vi "SLM Control.vi"() -> ()   [LabVIEW 2018]
uses:
  Controls/General Setting.ctl
  Controls/Buttons/Running Button.ctl
  Controls/Holo Setting.ctl
  Controls/Zernike Polynominals.ctl
  Controls/Buttons/Save Button.ctl
  Controls/Buttons/Load Button.ctl
  <vilib>/Utility/xml.llb/Read From XML File(string).vi
  <vilib>/Utility/xml.llb/Write to XML File(string).vi
panel:
  in  "Exit":bool
  in  "Load":T1
  in  "Save":T2
  in  "Holo 1 (Doughnut)":T3
  in  "Holo 0 (Z)":T3
  in  "General Setting":T6 {"Mode Matrix" items=["Name", "Sequence"]}
  out "Intensity Graph":u8[][](graph)
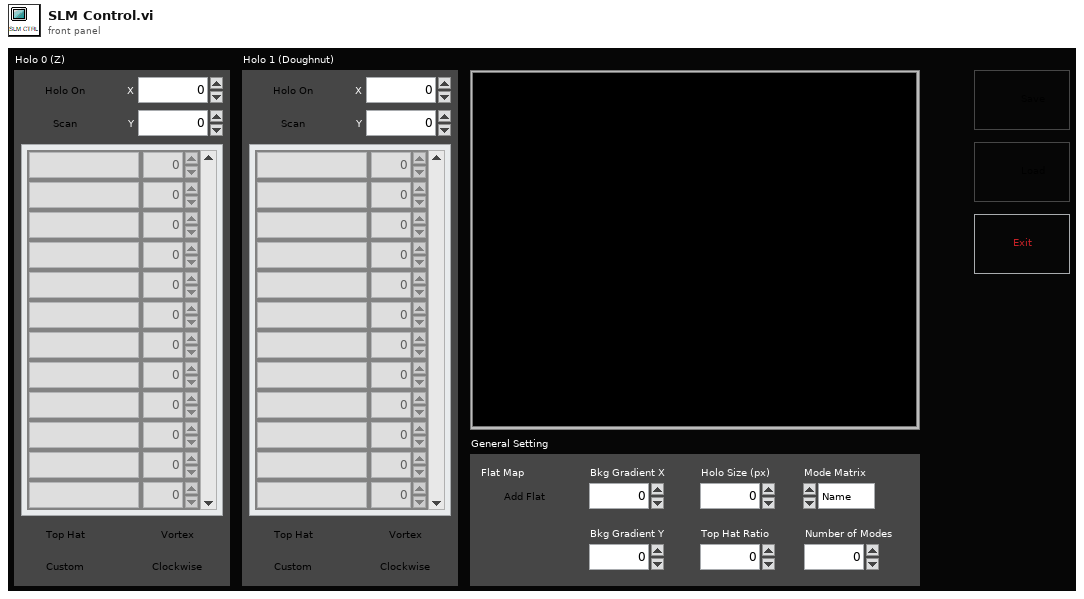
[diagram p1: front panel]
types:
  T1 = typedef "Load Button.ctl" = bool
  T2 = typedef "Save Button.ctl" = bool
  T3 = typedef "Holo Setting.ctl" = cluster{"Holo On":T4, "Scan":T4, "X":i16, "Y":i16, "Zernike Polynominals":T5, "Top Hat":T4, "Vortex":T4, "Clockwise":T4, "Custom":T4}
  T4 = typedef "Running Button.ctl" = bool
  T5 = typedef "Zernike Polynominals.ctl" = cluster{"Aberration Name":string, "Numeric":dbl}[]
  T6 = typedef "General Setting.ctl" = cluster{"Flat Map":T4, "Bkg Gradient X":dbl, "Bkg Gradient Y":dbl, "Holo Size (px)":i32, "Top Hat Ratio":dbl, "Number of Modes":i8, "Mode Matrix":u16}
  T7 = cluster{"Flat Map":T4, "Bkg Gradient X":bool, "Bkg Gradient Y":bool, "Holo Size (px)":bool, "Top Hat Ratio":bool, "Number of Modes":bool, "Mode Matrix":bool}
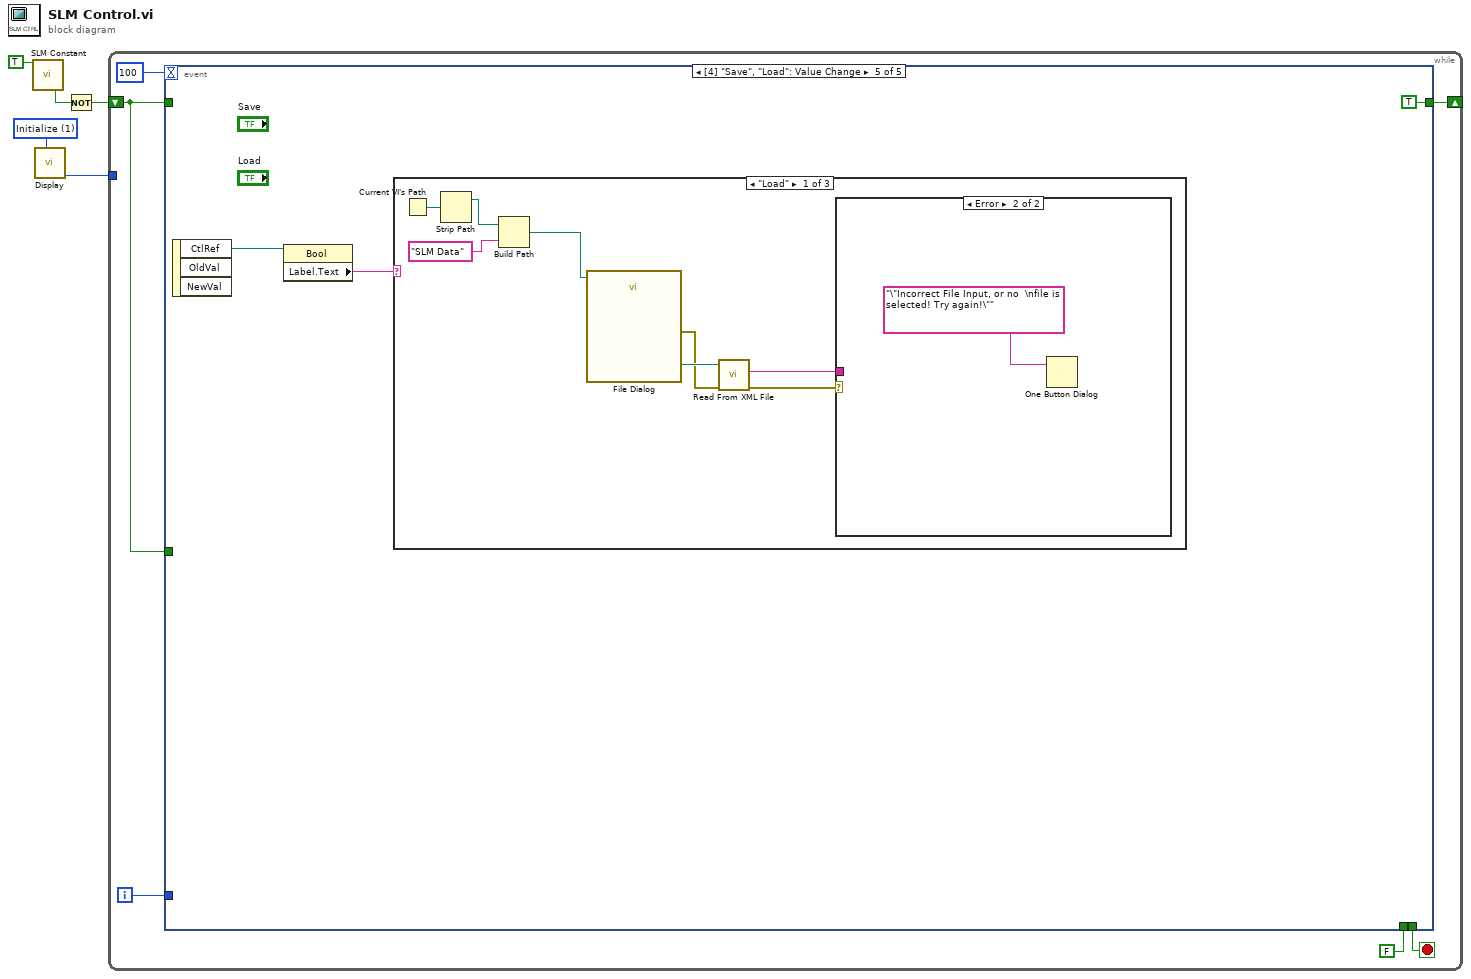
[diagram p0: block diagram]
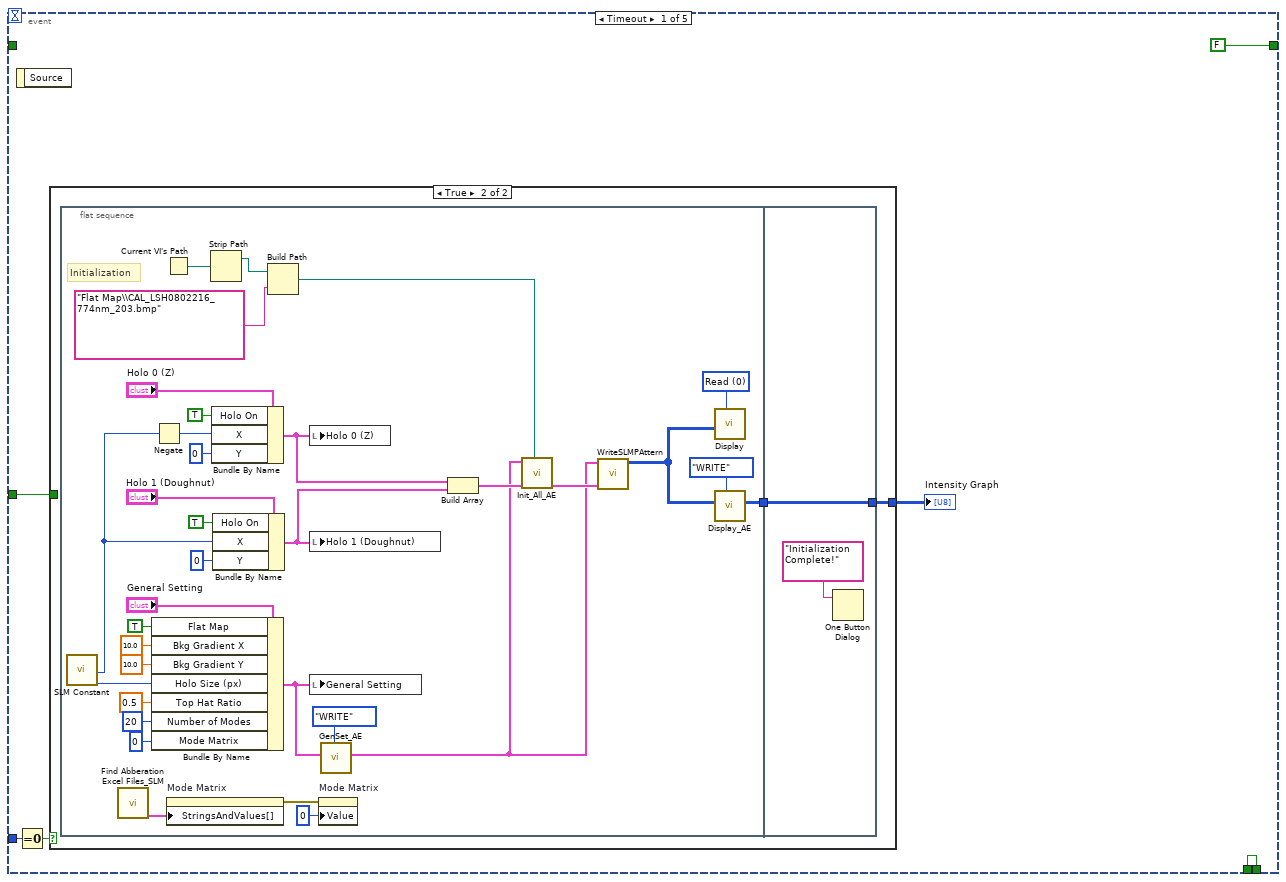
[diagram p2: hidden frame]
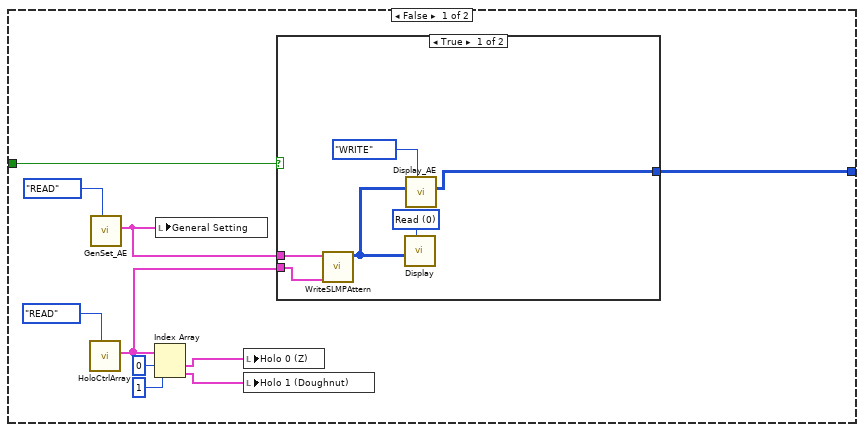
[diagram p3: hidden frame]
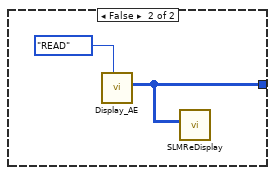
[diagram p4: hidden frame]
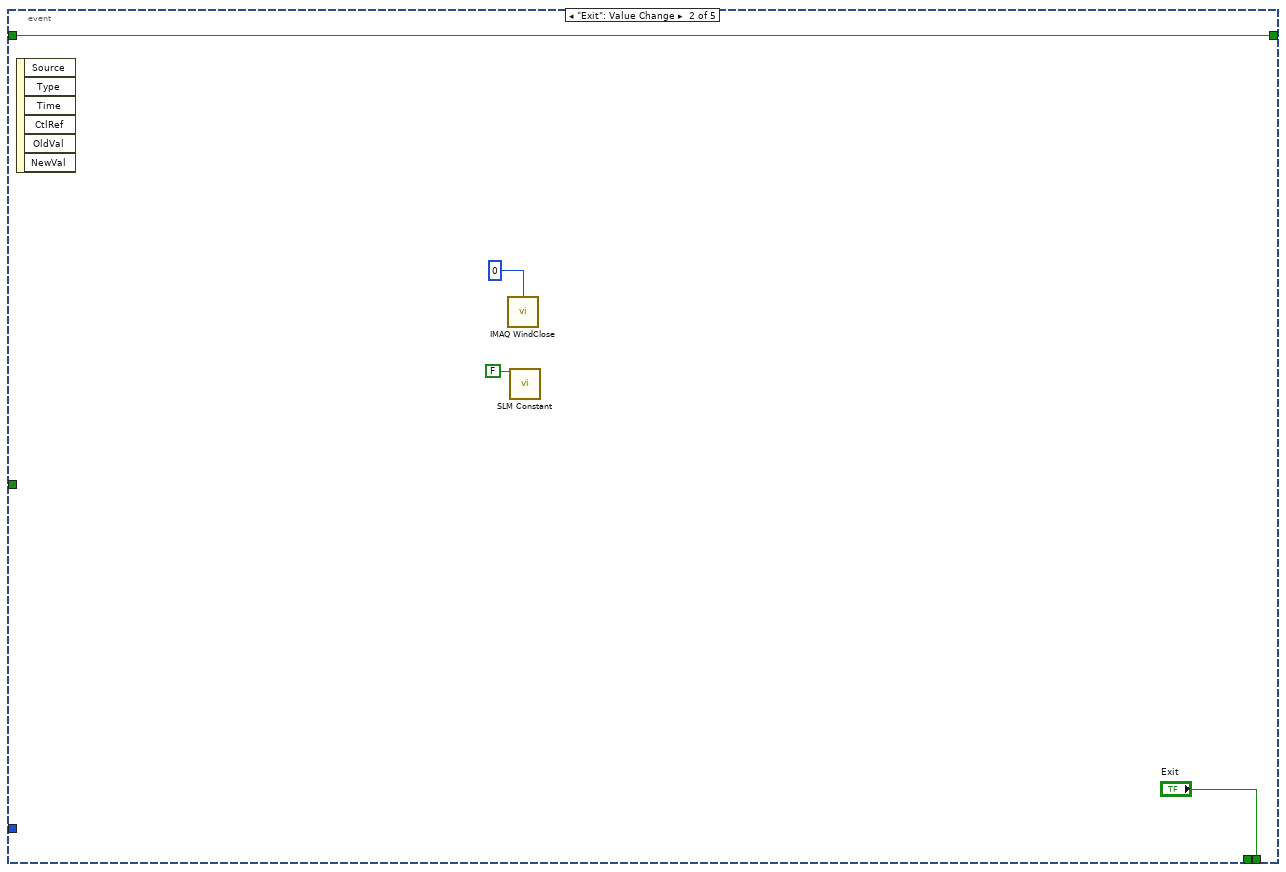
[diagram p5: hidden frame]
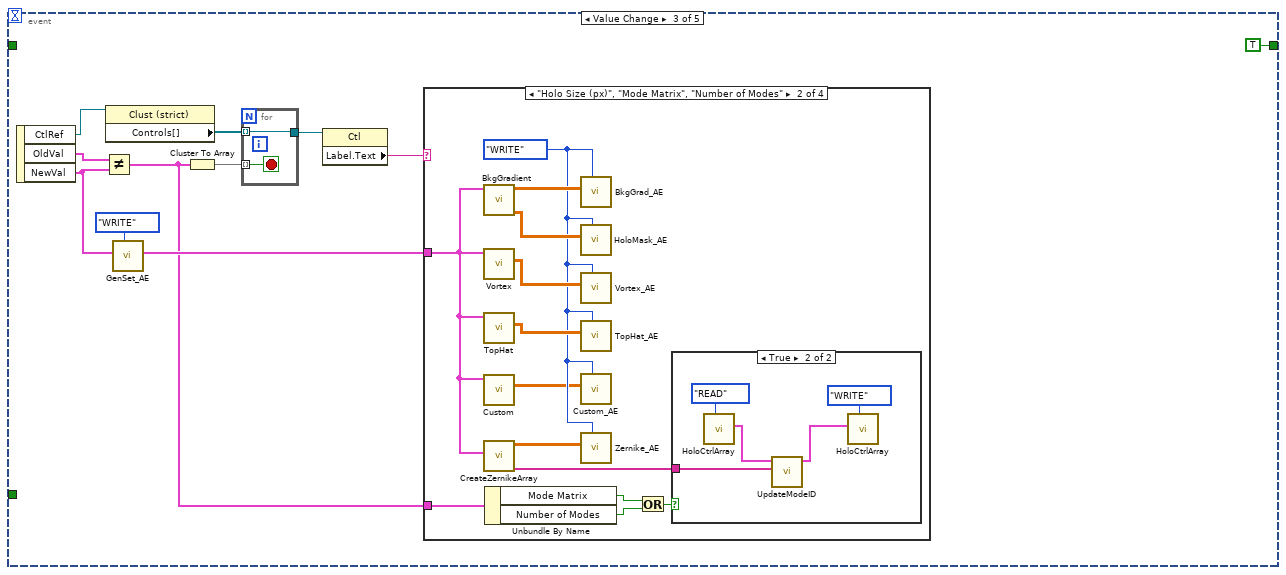
[diagram p6: hidden frame]
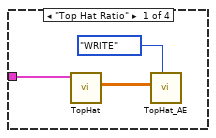
[diagram p7: hidden frame]
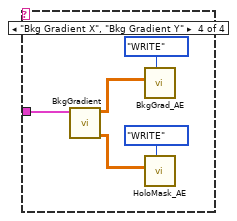
[diagram p10: hidden frame]
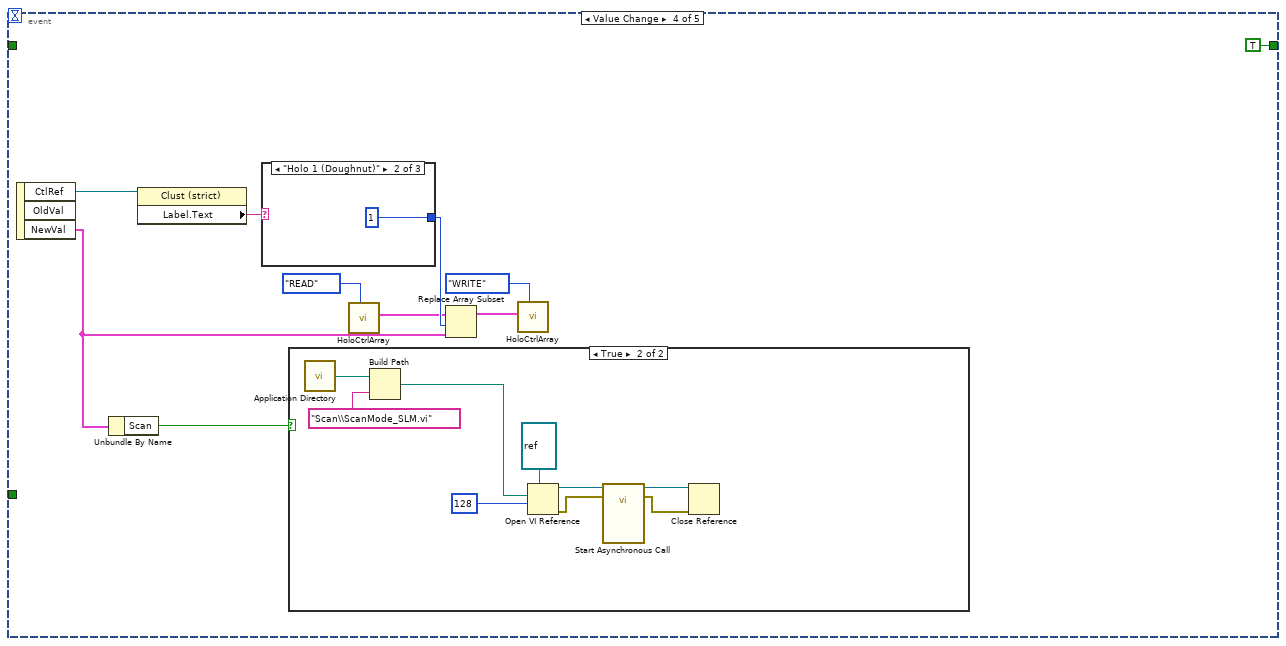
[diagram p11: hidden frame]
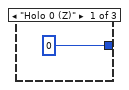
[diagram p13: hidden frame]
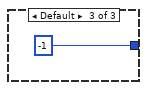
[diagram p14: hidden frame]
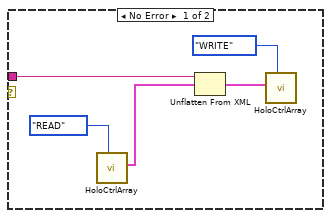
[diagram p15: hidden frame]
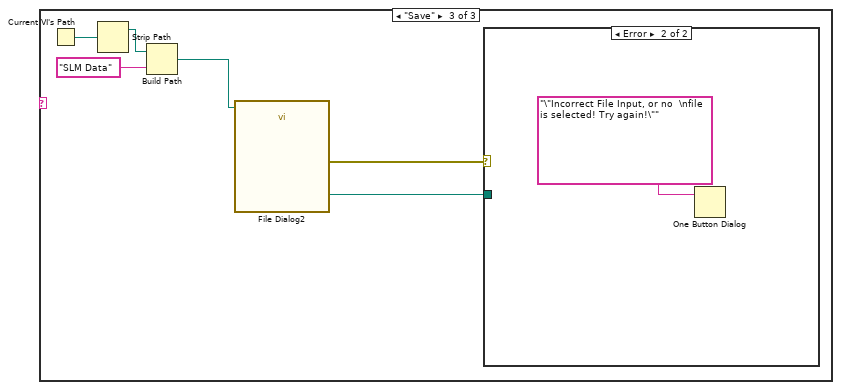
[diagram p17: hidden frame]
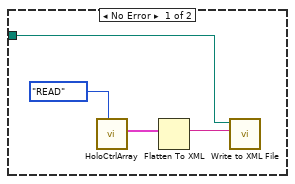
[diagram p18: hidden frame]
diagram:
  w2 = u16 1 items=["Read", "Initialize"] ("Action")
  n1 = call "SLM Constant.vi"("Ini. Mark In"=TRUE) -> ("Ini. Mark Out"=w4:bool)  [unwired: 9 in, 9 out]
  n2 = call "Display.vi"("Action"=w2) -> ("Read action"=w1:u16)  [unwired: 10 in]
  n3 = Not(x=w4) -> (.not. x?=w3:bool)
  n4 = while {
    shift-right: [w11] -> _
    shift-left: w3 -> [w6]
    tunnel: w1 -> [_]
    i -> [w7]
    stop <- w8 stop-if-true
    n5 = event shown="[4] \"Save\", \"Load\": Value Change" {
      selector: _ -> [_ _ _ _ _]
      dyn-events: _ -> [_ _ _ _ _]
      timeout: 100 -> [_ _ _ _ _]
      tunnel: [FALSE w76 TRUE TRUE TRUE] -> w11
      tunnel: FALSE -> [w16 _ _ _ _]
      tunnel: [w16 "Exit" _ _ _] -> w8
      tunnel: w7 -> [w15 _ _ _ _]
      tunnel: w6 -> [w13 _ _ _ _]
      tunnel: w6 -> [_ w76 _ _ _]
      event Timeout {
        n6 = event-data() -> ()  [unwired: 1 in, 1 out]
        n7 = Equal To 0?(x=w15) -> (x = 0?=w14:bool)
        n8 = case shown="True" w14 {
          tunnel: [w27 w37] -> w12
          tunnel: w13 -> [w26 _]
          frame False {
            n9 = call "HoloCtrlArray.vi"("Action"=enum16{"READ", "WRITE"}."READ") -> ("Holo Array Out"=w20:T3[])  [unwired: 10 in]
            n10 = call "GenSet_AE.vi"("Enum"=enum16{"READ", "WRITE"}."READ") -> ("General settings Out"=w24:T6)  [unwired: 10 in]
            n11 = Index Array(array=w20, index #1=0 ("index"), index #2=1 ("index")) -> (element #1=w19:T3, element #2=w18:T3)
            n12 = local write "General Setting"(w24) -> ()
            n13 = local write "Holo 0 (Z)"(w19) -> ()
            n14 = local write "Holo 1 (Doughnut)"(w18) -> ()
            n15 = case shown="True" w26 {
              tunnel: [w30 w34] -> w27
              tunnel: w24 -> [w33 _]
              tunnel: w20 -> [w32 _]
              frame True {
                w29 = u16 0 items=["Read", "Initialize"] ("Action")
                n16 = call "WriteSLMPAttern.vi"("Holo Array"=w32, "General settings"=w33) -> ("Display Array"=w28:u8[][])  [unwired: 9 in]
                n17 = call "Display.vi"("Action"=w29, "displayed matrix"=w28) -> ()  [unwired: 9 in, 1 out]
                n18 = call "Display_AE.vi"("Action"=enum16{"READ", "WRITE"}."WRITE", "Display Array In"=w28) -> ("Display Array Out"=w30:u8[][])  [unwired: 9 in]
              }
              frame False {
                n19 = call "Display_AE.vi"("Action"=enum16{"READ", "WRITE"}."READ") -> ("Display Array Out"=w34:u8[][])  [unwired: 10 in]
                n20 = call "SLMReDisplay.vi"("displayed matrix"=w34) -> ()  [unwired: 11 in]
              }
            }
          }
          frame True {
            n21 = flat-sequence {
              tunnel: [w40] -> w36
              tunnel: [w73] -> w37
              tunnel: w36 -> [w73]
              frame #0 {
                w43 = u16 0 items=["Read", "Initialize"] ("Action")
                # "Initialization"
                n22 = call "SLM Constant.vi"() -> ("Hologram Coordinate X"=w51:i32, "Hologram Size (px)"=w53:i32)  [unwired: 10 in, 8 out]
                n23 = call "Find Abberation Excel Files_SLM.vi"() -> ("Ring Menu"=w64:cluster{"result string":string, i32}[])  [unwired: 10 in, 1 out]
                n24 = Bundle By Name(cluster="General Setting", "Flat Map"=T4 TRUE, "Bkg Gradient X"=10.0, "Bkg Gradient Y"=10.0, "Holo Size (px)"=w53, "Top Hat Ratio"=0.5, "Number of Modes"=i8 20, "Mode Matrix"=u16 0) -> (w50:T6)
                n25 = Negate(x=w51) -> (-x=w52:i32)
                n26 = Current VI's Path() -> (path=w39:path)
                n27 = property on="Mode Matrix" class="Ring (strict)"("StringsAndValues[]"=w64) -> (error out=w63:errorcluster)  [unwired: 2 in, 1 out]
                n28 = Strip Path(path=w39) -> (stripped path=w38:path)  [unwired: 1 out]
                n29 = Bundle By Name(cluster="Holo 0 (Z)", "Holo On"=T4 TRUE, "X"=w52, "Y"=i16 0) -> (w55:T3)
                n30 = Bundle By Name(cluster="Holo 1 (Doughnut)", "Holo On"=T4 TRUE, "X"=w51, "Y"=i16 0) -> (w54:T3)
                n31 = Build Path(base path=w38, name or relative path="Flat Map\\CAL_LSH0802216_774nm_203.bmp") -> (appended path=w47:path)
                n32 = local write "Holo 0 (Z)"(w55) -> ()
                n33 = local write "Holo 1 (Doughnut)"(w54) -> ()
                n34 = local write "General Setting"(w50) -> ()
                n35 = property on="Mode Matrix" class="Ring (strict)"(error in=w63, "Value"=u16 0) -> ()  [unwired: 1 in, 2 out]
                n36 = call "GenSet_AE.vi"("Enum"=enum16{"READ", "WRITE"}."WRITE", "General settings"=w50) -> ("General settings Out"=w44:T6)  [unwired: 9 in]
                n37 = Build Array(w55, w54) -> (w46:T3[])
                n38 = call "Init_All_AE.vi"("Flat File Path"=w47, "HoloArray In"=w46, "General Setting"=w44) -> ("Holo Array Out"=w45:T3[])  [unwired: 8 in]
                n39 = call "WriteSLMPAttern.vi"("Holo Array"=w45, "General settings"=w44) -> ("Display Array"=w41:u8[][])  [unwired: 9 in]
                n40 = call "Display.vi"("Action"=w43, "displayed matrix"=w41) -> ()  [unwired: 9 in, 1 out]
                n41 = call "Display_AE.vi"("Action"=enum16{"READ", "WRITE"}."WRITE", "Display Array In"=w41) -> ("Display Array Out"=w40:u8[][])  [unwired: 9 in]
              }
              frame #1 {
                n42 = One Button Dialog(message="Initialization Complete!") -> ()  [unwired: 1 in, 1 out]
              }
            }
          }
        }
        "Intensity Graph" <- w12
      }
      event "Exit": Value Change {
        n43 = event-data() -> ()  [unwired: 1 in, 6 out]
        n44 = call "IMAQ WindClose"("Window Number (0...15)"=0) -> ()  [unwired: 2 in, 4 out]
        n45 = call "SLM Constant.vi"("Ini. Mark In"=FALSE) -> ()  [unwired: 9 in, 10 out]
      }
      event Value Change {
        n46 = event-data() -> ("CtlRef"=w88:refnum<vi>, "OldVal"=w86:T6, "NewVal"=w83:T6)  [unwired: 1 in]
        n47 = Not Equal?(x=w86, y=w83) -> (x != y?=w78:T7)
        n48 = property class="Clust (strict)"(reference=w88) -> ("Controls[]"=w87:refnum<vi>[])  [unwired: 1 in, 2 out]
        n49 = call "GenSet_AE.vi"("Enum"=enum16{"READ", "WRITE"}."WRITE", "General settings"=w83) -> ("General settings Out"=w79:T6)  [unwired: 9 in]
        n50 = Cluster To Array(cluster=w78) -> (array=w85:T4[])
        n51 = for {
          tunnel: [w116] -> w84
          tunnel: w87 -> [w116] mode=indexing
          tunnel: w85 -> [w115] mode=indexing
          stop <- w115 stop-if-true
        }
        n52 = property class="Ctl"(reference=w84) -> ("Label.Text"=w81:string)  [unwired: 1 in, 2 out]
        n53 = case shown="\"Holo Size (px)\", \"Mode Matrix\", \"Number of Modes\"" w81 {
          tunnel: w79 -> [w91 w94 _ w114]
          tunnel: w78 -> [_ w103 _ _]
          frame "Top Hat Ratio" {
            n54 = call "TopHat.vi"("General settings"=w91) -> ("TopHat"=w90:dbl[][])  [unwired: 10 in]
            n55 = call "TopHat_AE.vi"("Action"=enum16{"READ", "WRITE"}."WRITE", "TopHat In"=w90) -> ()  [unwired: 9 in, 1 out]
          }
          frame "Holo Size (px)", "Mode Matrix", "Number of Modes" {
            w93 = enum16{"READ", "WRITE"}."WRITE" ("Action")
            n56 = call "BkgGradient.vi"("General settings"=w94) -> ("Holo mask"=w97:dbl[][], "gradient"=w98:dbl[][])  [unwired: 9 in]
            n57 = call "Vortex.vi"("General settings"=w94) -> ("Vortex"=w96:dbl[][])  [unwired: 10 in]
            n58 = call "TopHat.vi"("General settings"=w94) -> ("TopHat"=w95:dbl[][])  [unwired: 10 in]
            n59 = call "Custom.vi"("General settings"=w94) -> ("Vortex"=w92:dbl[][])  [unwired: 10 in]
            n60 = call "CreateZernikeArray.vi"("General settings"=w94) -> ("Mode IDs"=w99:string[], "Modes Out"=w104:dbl[][][])  [unwired: 9 in]
            n61 = Unbundle By Name(w103) -> ("Mode Matrix"=w101:bool, "Number of Modes"=w102:bool)
            n62 = call "BkgGrad_AE.vi"("Action"=w93, "BkgGrad In"=w98) -> ()  [unwired: 9 in, 1 out]
            n63 = call "HoloMask_AE.vi"("Action"=w93, "HoloMask In"=w97) -> ()  [unwired: 9 in, 1 out]
            n64 = call "Vortex_AE.vi"("Action"=w93, "Vortex In"=w96) -> ()  [unwired: 9 in, 1 out]
            n65 = call "TopHat_AE.vi"("Action"=w93, "TopHat In"=w95) -> ()  [unwired: 9 in, 1 out]
            n66 = call "Custom_AE.vi"("Action"=w93, "Custom In"=w92) -> ()  [unwired: 9 in, 1 out]
            n67 = call "Zernike_AE.vi"("Action"=w93, "Zernike In"=w104) -> ()  [unwired: 9 in, 1 out]
            n68 = Or(x=w101, y=w102) -> (x .or. y?=w100:bool)
            n69 = case shown="True" w100 {
              tunnel: w99 -> [_ w108]
              frame False {
              }
              frame True {
                n70 = call "HoloCtrlArray.vi"("Action"=enum16{"READ", "WRITE"}."READ") -> ("Holo Array Out"=w107:T3[])  [unwired: 10 in]
                n71 = call "UpdateModeID.vi"("Mode IDs"=w108, "Array in"=w107) -> ("Array out"=w105:T3[])  [unwired: 9 in]
                n72 = call "HoloCtrlArray.vi"("Action"=enum16{"READ", "WRITE"}."WRITE", "Holo Array In"=w105) -> ()  [unwired: 9 in, 1 out]
              }
            }
          }
          frame Default {
          }
          frame "Bkg Gradient X", "Bkg Gradient Y" {
            n73 = call "BkgGradient.vi"("General settings"=w114) -> ("Holo mask"=w112:dbl[][], "gradient"=w113:dbl[][])  [unwired: 9 in]
            n74 = call "BkgGrad_AE.vi"("Action"=enum16{"READ", "WRITE"}."WRITE", "BkgGrad In"=w113) -> ()  [unwired: 9 in, 1 out]
            n75 = call "HoloMask_AE.vi"("Action"=enum16{"READ", "WRITE"}."WRITE", "HoloMask In"=w112) -> ()  [unwired: 9 in, 1 out]
          }
        }
      }
      event Value Change {
        n76 = event-data() -> ("CtlRef"=w126:refnum<vi>, "NewVal"=w118:T3)  [unwired: 1 in, 1 out]
        n77 = Unbundle By Name(w118) -> ("Scan"=w117:T4)
        n78 = property class="Clust (strict)"(reference=w126) -> ("Label.Text"=w125:string)  [unwired: 1 in, 2 out]
        n79 = case shown="\"Holo 1 (Doughnut)\"" w125 {
          tunnel: [0 1 -1] -> w123
          frame "Holo 0 (Z)" {
          }
          frame "Holo 1 (Doughnut)" {
          }
          frame Default {
          }
        }
        n80 = case shown="True" w117 {
          frame False {
          }
          frame True {
            n81 = call <vilib>:"Application Directory.vi"() -> ("Application Directory"=w133:path)
            n82 = Build Path(base path=w133, name or relative path="Scan\\ScanMode_SLM.vi") -> (appended path=w131:path)
            n83 = Open VI Reference(type specifier VI Refnum (for type only)=refnum<vi> refnum, vi path=w131, options=128) -> (vi reference=w130:refnum<vi>, error out=w129:errorcluster)  [unwired: 3 in]
            n84 = call-by-ref "Start Asynchronous Call"(reference=w130, error in=w129) -> (reference out=w128:refnum<vi>, error out=w127:errorcluster)  [unwired: 12 in]
            n85 = Close Reference(reference=w128, error in (no error)=w127) -> ()  [unwired: 1 out]
          }
        }
        n86 = call "HoloCtrlArray.vi"("Action"=enum16{"READ", "WRITE"}."READ") -> ("Holo Array Out"=w122:T3[])  [unwired: 10 in]
        n87 = Replace Array Subset(array=w122, new element=w118, index=w123) -> (w120:T3[])
        n88 = call "HoloCtrlArray.vi"("Action"=enum16{"READ", "WRITE"}."WRITE", "Holo Array In"=w120) -> ()  [unwired: 9 in, 1 out]
      }
      event Value Change {
        n89 = event-data() -> ("CtlRef"=w141:refnum<vi>)  [unwired: 1 in, 2 out]
        n90 = property class="Bool"(reference=w141) -> ("Label.Text"=w140:string)  [unwired: 1 in, 2 out]
        n91 = case shown="\"Load\"" w140 {
          frame "Load" {
            n92 = Current VI's Path() -> (path=w143:path)
            n93 = Strip Path(path=w143) -> (stripped path=w142:path)  [unwired: 1 out]
            n94 = Build Path(base path=w142, name or relative path="SLM Data") -> (appended path=w145:path)
            n95 = call "File Dialog"("start path"=w145) -> ("selected path"=w149:path, "error out"=w148:errorcluster)  [unwired: 11 in, 2 out]
            n96 = call-poly <vilib>:"Read From XML File.vi"("error in (no error)"=w148, "XML File Path"=w149) -> ("error out"=w147:errorcluster, "XML Elements"=w146:string)  [unwired: 7 in, 1 out]
            n97 = case shown="Error" w147 {
              tunnel: w146 -> [w154 _]
              frame No Error {
                n98 = call "HoloCtrlArray.vi"("Action"=enum16{"READ", "WRITE"}."READ") -> ("Holo Array Out"=w153:T3[])  [unwired: 10 in]
                n99 = Unflatten From XML(xml string=w154, type=w153) -> (value=w151:T3[])  [unwired: 1 in, 1 out]
                n100 = call "HoloCtrlArray.vi"("Action"=enum16{"READ", "WRITE"}."WRITE", "Holo Array In"=w151) -> ()  [unwired: 9 in, 1 out]
              }
              frame Error {
                n101 = One Button Dialog(message="\"Incorrect File Input, or no  \nfile is selected! Try again!\"") -> ()  [unwired: 1 in, 1 out]
              }
            }
          }
          frame Default {
          }
          frame "Save" {
            n102 = Current VI's Path() -> (path=w157:path)
            n103 = Strip Path(path=w157) -> (stripped path=w156:path)  [unwired: 1 out]
            n104 = Build Path(base path=w156, name or relative path="SLM Data") -> (appended path=w161:path)
            n105 = call "File Dialog2"("start path"=w161) -> ("selected path"=w158:path, "error out"=w159:errorcluster)  [unwired: 11 in, 2 out]
            n106 = case shown="Error" w159 {
              tunnel: w158 -> [w163 _]
              frame No Error {
                n107 = call "HoloCtrlArray.vi"("Action"=enum16{"READ", "WRITE"}."READ") -> ("Holo Array Out"=w164:T3[])  [unwired: 10 in]
                n108 = Flatten To XML(anything=w164) -> (xml string=w162:string)
                n109 = call-poly <vilib>:"Write to XML File.vi"("XML Input"=w162, "XML File Path"=w163) -> ()  [unwired: 7 in, 3 out]
              }
              frame Error {
                n110 = One Button Dialog(message="\"Incorrect File Input, or no  \nfile is selected! Try again!\"") -> ()  [unwired: 1 in, 1 out]
              }
            }
          }
        }
      }
    }
  }
